vi "GEA3 Board ID to Board Index.vi"(0 "GEA3 Serial Number":string, 11 "Error In":errorcluster) -> (4 "Board Found?":bool, 6 "Report Text":string="Board not found.", 8 "Board Index":i32=-1, 10 "Boards Found":string[](array[string]), 15 "Error Out":errorcluster)   [LabVIEW 2019, in "GEA2_Toolkit.lvlib"]
uses:
  library/GEA2_Toolkit.lvlib
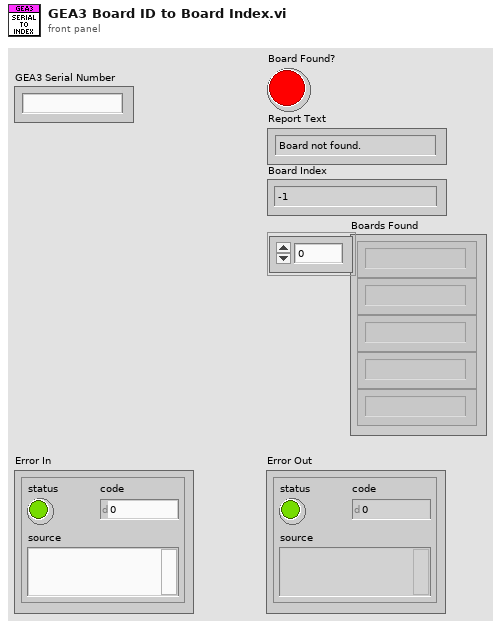
[diagram p1: front panel]
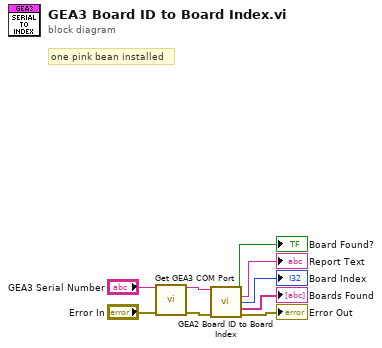
[diagram p0: block diagram]
diagram:
  # "one pink bean installed"
  n1 = call "Get GEA3 COM Port.vi"("GEA3 Serial Number"="GEA3 Serial Number", "Error In"="Error In") -> ("GEA3 COM Port"=w9:string, "Error Out"=w8:errorcluster)  [unwired: 12 in]
  n2 = call "GEA2 Board ID to Board Index.vi"("Board ID"=w9, "Error In"=w8) -> ("Board Found?"=→"Board Found?":bool, "Report Text"=→"Report Text":string, "Board Index"=→"Board Index":i32, "Boards Found"=→"Boards Found":string[], "Error Out"=→"Error Out":errorcluster)  [unwired: 9 in]
